vi "ConfigureOutputTrigger.vi"(0 "object in":refnum<class "Hamamatsu_simulated.lvclass">, 2 "Trigger Output Settins":T1={"Output Trigger Type"={"Mode"=1, "Polarity"=1}, "Programmable Options"={"Width"=0.003, "Delay"=0.0, "Source"=2}, "Port"=1} {"Output Trigger Type"."Mode" items=["Low"=1, "Global Exposure"=2, "Programmable"=3, "Trigger Ready"=4, "High"=5]; "Output Trigger Type"."Polarity" items=["Negative"=1, "Positive"=2]; "Programmable Options"."Source" items=["Exposure"=1, "Readout End"=2, "V Sync"=3, "H Sync"=4, "Trigger"=6]}, 5 "error in (no error)":errorcluster) -> (14 "object out":refnum<class "Hamamatsu_simulated.lvclass">, 19 "error out":errorcluster)   [LabVIEW 2024, in "Hamamatsu_simulated.lvclass"]
uses:
  Hamamatsu_simulated.lvclass
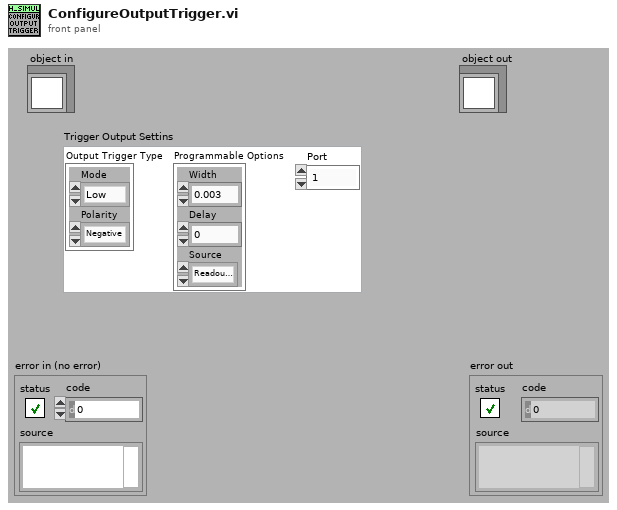
[diagram p1: front panel]
types:
  T1 = cluster{"Output Trigger Type":cluster{"Mode":u32, "Polarity":u32}, "Programmable Options":cluster{"Width":dbl, "Delay":dbl, "Source":u32}, "Port":i32}
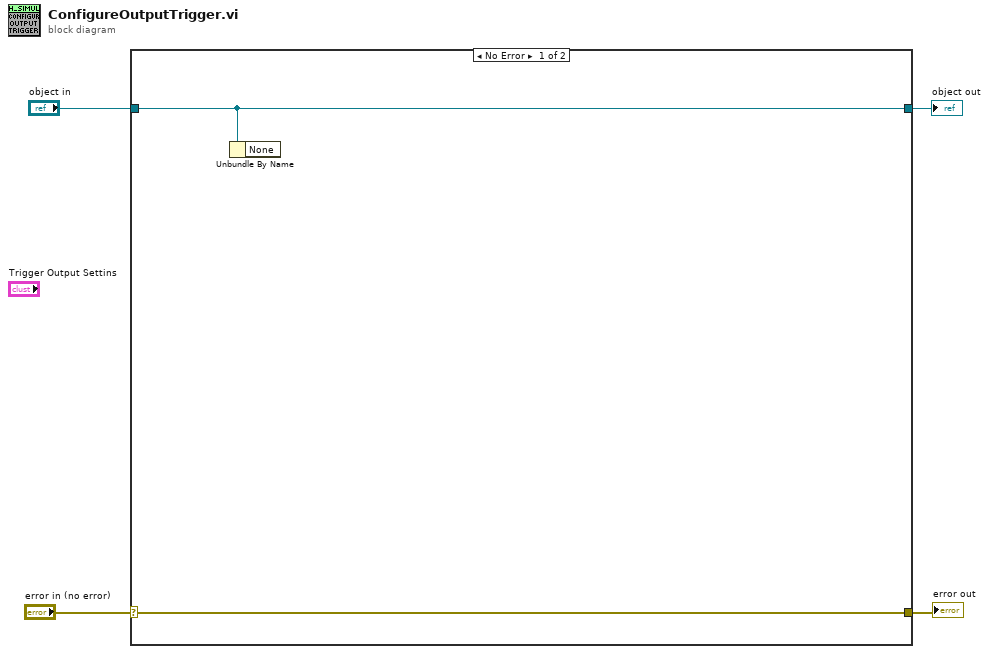
[diagram p0: block diagram]
diagram:
  n1 = case shown="No Error" "error in (no error)" {
    selector: "error in (no error)" -> [w6 w8]
    tunnel: [w6 w8] -> w3
    tunnel: [w5 w7] -> w1
    tunnel: "object in" -> [w5 w7]
    frame No Error {
      n2 = Unbundle By Name(w5) -> ()  [unwired: 1 out]
    }
    frame Error {
    }
  }
  "error out" <- w3
  "object out" <- w1
